vi "Werte sammeln.vi"() -> (2 "Temperatur":sgl, 3 "Druck FTIR":sgl)   [LabVIEW 2020, in "EPA 1065.lvlib" / "Dichtheitstest 1065-345.lvlib"]
uses:
  Dichtheitstest 1065-345.lvlib
  Seiten/Anlagengrenzwerte/FGV Anlagengrenzwerte Aktionen.ctl
  cRIO/PC/Kommunikation mit cRIO.lvlib
  Allgemein/allgemeine Sub-VIs.lvlib
  Seiten/Anlagengrenzwerte/Anlagengrenzwerte.lvlib
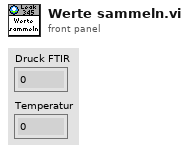
[diagram p1: front panel]
types:
  T1 = typedef "Anlagengrenzwerte.lvlib/FGV Anlagengrenzwerte Aktionen.ctl" = enum16{"Lesen", "Grenzwerte schreiben"}
  T2 = typedef "Anlagengrenzwerte.lvlib/Anlagen-Grenzwerte Anzeige.ctl" = cluster{"Eingangsdruck FT-IR:":T3, "Durchfluss FT-IR:":T3, "Durchfluss CalGas:":T3, "Druck Ausgang:":T3, "Druck Kalter Block:":T3, "Heizleitungen intern:":T3, "Heizleitung zu FT-IR:":T3, "Heizung Filterblock:":T3, "Heizung Pumpe:":T3, "Heizleitung Extern SP1:":T3, "Heizleitung Extern SP2:":T3, "FT-IR Heizung Messzelle:":T3, "Schaltschranktemperatur:":T3, "Gaskühler:":T3}
  T3 = typedef "Anlagengrenzwerte.lvlib/Anlagen-Parameter Anzeige.ctl" = cluster{"Sollwert":sgl, "Warn-Min":sgl, "Warn-Max":sgl, "Abschalt-Min":sgl, "Abschalt-Max":sgl, "Regler":u16}
  T4 = typedef "Verwaltung - cRIO.lvlib/Analog Eingaenge.ctl" = cluster{"AI0: Durchfluss FT-IR":sgl, "AI1: Druck Ausgang":sgl, "AI2: Umgebungsdruck":sgl, "AI3: Druck FT-IR":sgl, "AI4: Druck CalGas":sgl, "AI5: Reserve":sgl, "AI6: Reserve":sgl, "AI7: Reserve":sgl, "Rohwert Durchfluss FT-IR":sgl, "Rohwert Druck Ausgang":sgl, "Rohwert Umgebungsdruck":sgl, "Rohwert Druck FT-IR":sgl, "Rohwert Druck CalGas":sgl, "Rohwert AI5":sgl, "Rohwert AI6":sgl, "Rohwert AI7":sgl, "Rohwert Diffdruck mbar FTIR":sgl}
  T5 = typedef "Verwaltung - cRIO.lvlib/TC Eingaenge.ctl" = cluster{"TC0: Reserve":sgl, "TC1: HL zu FT-IR":sgl, "TC2: HL Extern SP1":sgl, "TC3: HL Extern SP2":sgl, "TC4: Reserve":sgl, "TC5: Reserve":sgl, "TC6: Reserve":sgl, "TC7: Reserve":sgl, "TC8: FT-IR":sgl, "TC9: Reserve":sgl, "TC10: Schaltschrank":sgl, "TC11: Umgebung":sgl}
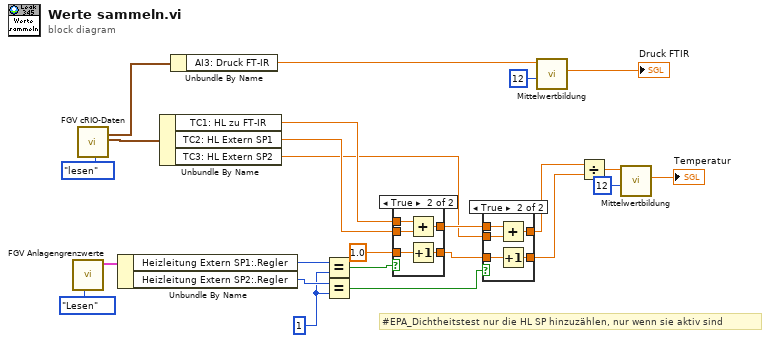
[diagram p0: block diagram]
diagram:
  w12 = u16 1 ("Heizleitung Extern:.Regler")
  # "#EPA_Dichtheitstest nur die HL SP hinzuzählen, nur wenn sie aktiv sind"
  n1 = call "FGV Anlagengrenzwerte.vi"("Aktion"=FGV_Anlagengrenzwerte_Aktionen."Lesen") -> ("Anlagen-Grenzwerte Anzeige"=w15:T2)  [unwired: 10 in]
  n2 = call "FGV cRIO-Daten.vi"("Aktion"=enum16{"lesen", "schreiben"}."lesen") -> ("Analog Input"=w17:T4, "TC Eingänge"=w1:T5)  [unwired: 9 in, 8 out]
  n3 = Unbundle By Name(w15) -> ("Heizleitung Extern SP1:.Regler"=w14:u16, "Heizleitung Extern SP2:.Regler"=w13:u16)
  n4 = Unbundle By Name(w1) -> ("TC1: HL zu FT-IR"=w11:sgl, "TC2: HL Extern SP1"=w8:sgl, "TC3: HL Extern SP2"=w6:sgl)
  n5 = Unbundle By Name(w17) -> ("AI3: Druck FT-IR"=w19:sgl)
  n6 = Equal?(x=w14, y=w12) -> (x = y?=w10:bool)
  n7 = Equal?(x=w13, y=w12) -> (x = y?=w5:bool)
  n8 = case shown="True" w10 {
    tunnel: sgl 1.0 ("y") -> [w25 w31]
    tunnel: w11 -> [w26 w30]
    tunnel: w8 -> [_ w29]
    tunnel: [w25 w28] -> w4
    tunnel: [w26 w27] -> w7
    frame False {
    }
    frame True {
      n9 = Add(x=w30, y=w29) -> (x+y=w27:sgl)
      n10 = Increment(x=w31) -> (x+1=w28:sgl)
    }
  }
  n11 = case shown="True" w5 {
    tunnel: w4 -> [w32 w38]
    tunnel: w7 -> [w33 w37]
    tunnel: w6 -> [_ w36]
    tunnel: [w32 w35] -> w3
    tunnel: [w33 w34] -> w2
    frame False {
    }
    frame True {
      n12 = Add(x=w37, y=w36) -> (x+y=w34:sgl)
      n13 = Increment(x=w38) -> (x+1=w35:sgl)
    }
  }
  n14 = call "Mittelwertbildung.vi"("Anzahl Werte"=u8 12, "Neuer Wert"=w19) -> ("gemittelter Wert"=→"Druck FTIR":sgl)  [unwired: 7 in, 2 out]
  n15 = Divide(x=w2, y=w3) -> (x/y=w23:sgl)
  n16 = call "Mittelwertbildung.vi"("Anzahl Werte"=u8 12, "Neuer Wert"=w23) -> ("gemittelter Wert"=→"Temperatur":sgl)  [unwired: 7 in, 2 out]
